vi "Metronome.vi"() -> ()   [LabVIEW 2011, in "Messenging.lvlib" / "Metronome.lvclass"]
uses:
  Metronome.lvclass
  Parallel Process.lvclass
  Interprocess Messenger/TextVarientMessage/MSG.lvclass
  Interprocess Messenger/Receiver/MGR (Receive type).lvclass
  ObserverRegister/ObserverRegistry.lvclass
  Interprocess Messenger/TextVarientMessage/Write (no data).vi
  Interprocess Messenger/TextVarientMessage/Write VarMessage.vi
  Interprocess Messenger/VarMessage/VarMessage.lvclass
panel:
  in  "Startup Message":refnum<class "MSG.lvclass">
  # "QueueMessenger Based"
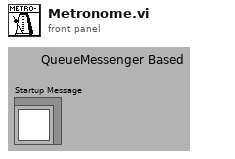
[diagram p1: front panel]
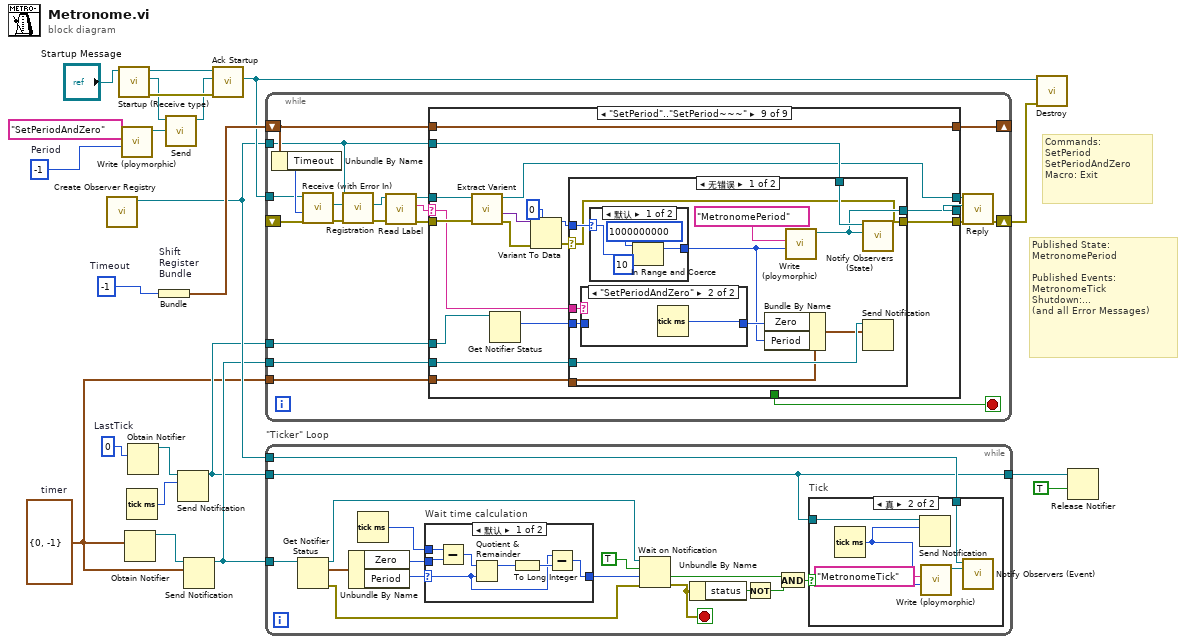
[diagram p0: block diagram]
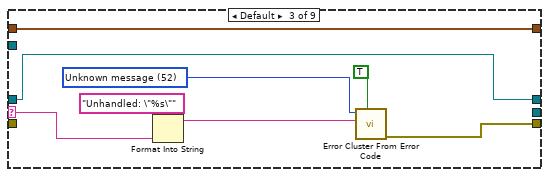
[diagram p6: hidden frame]
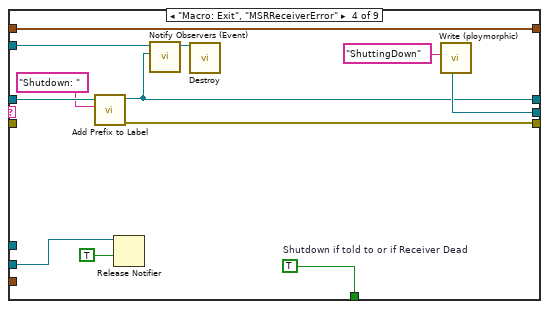
[diagram p7: hidden frame]
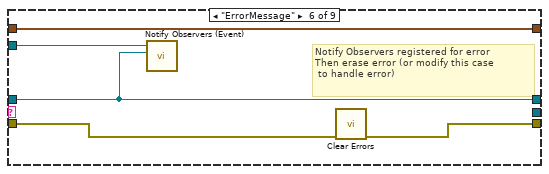
[diagram p9: hidden frame]
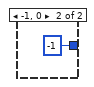
[diagram p12: hidden frame]
diagram:
  w2 = -1  # Period
  w11 = u32 0  # LastTick
  w4 = cluster{"Zero":u32, "Period":i32} {"Zero"=0, "Period"=-1}  # timer
  w19 = -1  # Timeout
  # "Published State:\nMetronomePeriod\n\nPublished Events:\nMetronomeTick\nShutdown:...\n(and all Error Messages)"
  # "Commands:\nSetPeriod\nSetPeriodAndZero\nMacro: Exit"
  n1 = call "Create Observer Registry.vi"() -> ("ObsReg"=w14:refnum<class "ObserverRegistry.lvclass">)  [unwired: 1 in, 10 out]
  n2 = call "Startup (Receive type).vi"("Startup Message"="Startup Message") -> ("error out"=w17:errorcluster, "Command Messenger out"=w6:refnum<class "MGR (Receive type).lvclass">, "Starup Message"=w22:refnum<class "MSG.lvclass">)  [unwired: 1 in, 7 out]
  n3 = call-poly "Write (ploymorphic).vi"("Varient"=w2, "Label"="SetPeriodAndZero") -> ("Message"=w1:refnum<class "VarMessage.lvclass">)  [unwired: 1 in, 8 out]
  n4 = Obtain Notifier(notification data type=w4) -> (notifier out=w15:refnum<notifier>)  [unwired: 2 in, 3 out]
  n5 = Tick Count (ms)() -> (millisecond timer value=w7:u32)
  n6 = Obtain Notifier(notification data type=w11) -> (notifier out=w12:refnum<notifier>)  [unwired: 2 in, 3 out]
  n7 = Bundle "Shift\nRegister\nBundle"("Timeout"=w19) -> (w18:cluster{"Timeout":i32})  [unwired: 1 in]
  n8 = call-dynamic "Send.vi"("Message"=w1, "MSR Parent in"=w6) -> ("MSR Parent out"=w5:refnum<class "MGR (Receive type).lvclass">)  [unwired: 1 in, 8 out]
  n9 = Send Notification(notification=w7, notifier=w12) -> (notifier out=w10:refnum<notifier>)  [unwired: 1 in, 1 out]
  n10 = Send Notification(notification=w4, notifier=w15) -> (notifier out=w13:refnum<notifier>)  [unwired: 1 in, 1 out]
  n11 = call "Ack Startup.vi"("error in"=w17, "Command Messenger"=w5, "Starup Message"=w22) -> ("Command Messenger"=w16:refnum<class "MGR (Receive type).lvclass">)  [unwired: 3 in, 5 out]
  n12 = while {
    shift-right: [w40] -> w20
    shift-left: _ -> [w43]
    shift-right: [w36] -> _
    shift-left: w18 -> [w35]
    tunnel: w16 -> [w34]
    tunnel: w14 -> [w26]
    tunnel: w13 -> [w24]
    tunnel: w10 -> [w25]
    tunnel: w4 -> [w23]
    stop <- w38 stop-if-true
    n13 = Unbundle By Name(w35) -> ("Timeout"=w37:i32)
    n14 = call-dynamic "Receive (with Error In).vi"("error in (no error)"=w43, "timeout in ms (5000)"=w37, "MGR in"=w34) -> ("error out"=w28:errorcluster, "Message"=w33:refnum<class "MSG.lvclass">)  [unwired: 7 out]
    n15 = call "Registration.vi"("error in (no error)"=w28, "Message"=w33, "ObserverRegistry in"=w26) -> ("error out"=w27:errorcluster, "Message (Register Commands filtered out)"=w32:refnum<class "MSG.lvclass">)  [unwired: 7 out]
    n16 = call-dynamic "Read Label.vi"("error in (no error)"=w27, "Message"=w32) -> ("error out"=w29:errorcluster, "Label"=w31:string, "Message"=w30:refnum<class "MSG.lvclass">)  [unwired: 7 out]
    n17 = case shown="\"SetPeriod\"..\"SetPeriod~~~\"" w31 {
      selector: w31 -> [_ _ w57 _ _ _ _ _ w86]
      tunnel: [w45 w47 w50 w60 w71 w73 w78 w81 w84] -> w39
      tunnel: [w44 w48 w51 w61 w70 w75 w79 w82 w89] -> w42
      tunnel: [_ _ _ w64 _ _ _ _ w90] -> w41
      tunnel: [_ _ _ w68 _ _ _ _ _] -> w38
      tunnel: [w46 w49 w52 w69 w72 w77 w80 w83 w92] -> w36
      tunnel: w35 -> [w46 w49 w52 w69 w72 w77 w80 w83 w92]
      tunnel: w30 -> [w44 w48 w51 w63 w70 w75 w79 w82 w97]
      tunnel: w29 -> [w45 w47 _ _ w71 w74 w78 w81 w96]
      tunnel: w26 -> [_ _ _ w66 _ w76 _ _ w91]
      tunnel: w25 -> [_ _ _ _ _ _ _ _ w94]
      tunnel: w24 -> [_ _ _ w58 _ _ _ _ w88]
      tunnel: w23 -> [_ _ _ _ _ _ _ _ w87]
      frame "------- Core (don't modify) --------" {
        # "Core Cases for template"
      }
      frame "<null> message (ignore)", "MSG" {
        # "\"Null\" Message --> Ignore these"
      }
      frame Default {
        w54 = 52 items=["No error", "Argument error", "Memory is full", "Out of zone", "End of file", "File already open", "Generic file I/O error", "File not found", "File permission error", "Disk is full", "Duplicate path", "Too many files open", "System feature not enabled", "Resource file not found", "Cannot add resource", "Resource not found", "Image not found", "Image memory error", "Pen does not exist", "Config type invalid", "Config token not found", "Config parse error", "Config memory error", "Bad external code format", "Bad external code offset", "External code not present", "Null window", "Destroy window error", "Null menu", "Print aborted", "Bad print record", "Print driver error", "Windows error during printing", "Memory error during printing", "Print dialog error", "Generic print error", "Invalid device refnum", "Device not found", "Device parameter error", "Device unit error", "Cannot open device", "Device call aborted", "Generic error", "Cancelled by user", "Object ID too low", "Object ID too high", "Object not in heap", "Unknown heap", "Unknown object (invalid DefProc)", "Unknown object (DefProc not in table)", "Message out of range", "Invalid (null) method", "Unknown message", "Manager call not supported", "Bad address", "Network operation in progress", "Network operation timed out", "Connection is busy", "Network attribute not supported", "Network error", "Address in use", "System out of memory", "Connection aborted", "Connection refused", "Not connected", "Already connected", "Connection closed", "Initialization error (interapplication manager)", "Bad occurrence", "Wait on unbound occurrence handler", "Occurrence queue overflow", "Datalog type conflict", "Unused", "Unrecognized type (interapplication manager)", "Memory corrupt", "Failed to make temporary DLL", "Old CIN version", "Drag socket not found", "Failed to load drop-object", "Failed to register OLE object", "Failed to release OLE object", "Format specifier type mismatch", "Unknown format specifier", "Too few format specifiers", "Too many format specifiers", "Scan failed", "Newer CIN version", "Error converting to variant", "Runtime menu error", "Password tampered", "Variant attribute not found", "Incompatible variant data type", "Event data is not available", "Event Store is not present", "Occurrence is not found", "Event Queue is not created", "Event info is not available", "Refnum passed is NULL", "Error retrieving Class GUID", "Error retrieving CoClass GUID", "Error retrieving TypeLib GUID.", "Bad built application magic bytes.", "Specific driver is different from the specific driver associated with the Logical Name.", "There is no session opened to the class driver.", "Max Error", "MAX - Error with config objects", "MAX - Error loading configuration", "MAX - Group not supported"]
        n18 = Format Into String(format string="Unhandled: \"%s\"", w57) -> (resulting string=w55:string)  [unwired: 2 in, 1 out]
        n19 = call <vilib>:"Error Cluster From Error Code.vi"("show call chain? (False)"=TRUE, "error message (\"\")"=w55, "error code (0)"=w54) -> ("error out"=w50:errorcluster)  [unwired: 1 in, 5 out]
      }
      frame "Macro: Exit", "MSRReceiverError" {
        w68 = TRUE  # Shutdown if told to or if Receiver Dead
        n20 = call-dynamic "Add Prefix to Label.vi"("Prefix to add"="Shutdown: ", "Message"=w63) -> ("error out"=w60:errorcluster, "Message"=w61:refnum<class "MSG.lvclass">)  [unwired: 1 in, 7 out]
        n21 = Release Notifier(notifier=w58, force destroy? (F)=TRUE) -> ()  [unwired: 1 in, 3 out]
        n22 = call "Notify Observers (Event).vi"("Message"=w61, "ObserverRegistry in"=w66) -> ("ObserverRegistry out"=w67:refnum<class "ObserverRegistry.lvclass">)  [unwired: 1 in, 8 out]
        n23 = call "Destroy.vi"("ObserverRegistry.lvclass in"=w67) -> ()  [unwired: 1 in, 10 out]
        n24 = call-poly "Write (ploymorphic).vi"("Label"="ShuttingDown") -> ("Message"=w64:refnum<class "MSG.lvclass">)  [unwired: 1 in, 9 out]
      }
      frame "-------- Core (modify to suit) -----" {
        # "Core Cases for template"
      }
      frame "ErrorMessage" {
        # "Notify Observers registered for error\nThen erase error (or modify this case\n to handle error)"
        n25 = call "Notify Observers (Event).vi"("Message"=w75, "ObserverRegistry in"=w76) -> ()  [unwired: 1 in, 9 out]
        n26 = call <vilib>:"Clear Errors.vi"("error in (no error)"=w74) -> ("error out"=w73:errorcluster)  [unwired: 6 out]
      }
      frame "MSRReceiveTimedOut" {
      }
      frame "-------- Metronome --------" {
      }
      frame "SetPeriod".."SetPeriod~~~" {
        n27 = call-dynamic "Extract Varient.vi"("error in (no error)"=w96, "Message"=w97) -> ("error out"=w99:errorcluster, "Varient"=w98:variant, "Message"=w89:refnum<class "MSG.lvclass">)  [unwired: 1 in, 6 out]
        n28 = Get Notifier Status(notifier=w94) -> (current notification=w93:u32)  [unwired: 1 in, 4 out]
        n29 = Variant To Data(error in=w99, type=0 ("Period"), Variant=w98) -> (data=w100:i32, error out=w85:errorcluster)
        n30 = case shown="无错误" w85 {
          selector: w85 -> [w101 w120]
          tunnel: w100 -> [w112 _]
          tunnel: w93 -> [w108 _]
          tunnel: w91 -> [w107 _]
          tunnel: [w106 _] -> w90
          tunnel: w88 -> [w105 _]
          tunnel: w87 -> [w103 _]
          tunnel: w86 -> [w102 _]
          tunnel: [w101 w120] -> w84
          frame No Error {
            n31 = case shown="\"SetPeriodAndZero\"" w102 {
              tunnel: w108 -> [w118 _]
              tunnel: [w118 w119] -> w111
              frame "SetPeriod", Default {
              }
              frame "SetPeriodAndZero" {
                n32 = Tick Count (ms)() -> (millisecond timer value=w119:u32)
              }
            }
            n33 = case shown="默认" w112 {
              selector: w112 -> [w113 _]
              tunnel: [w114 -1 ("upper limit")] -> w110
              frame Default {
                n34 = In Range and Coerce(upper limit=1000000000, x=w113, lower limit=10) -> (coerced(x)=w114:i32)  [unwired: 1 out]
              }
              frame -1, 0 {
              }
            }
            n35 = Bundle By Name(cluster=w103, "Zero"=w111, "Period"=w110) -> (w104:cluster{"Zero":u32, "Period":i32})
            n36 = call-poly "Write (ploymorphic).vi"("Varient"=w110, "Label"="MetronomePeriod") -> ("Message"=w106:refnum<class "VarMessage.lvclass">)  [unwired: 1 in, 8 out]
            n37 = call "Notify Observers (State).vi"("State Message"=w106, "ObserverRegistry in"=w107) -> ()  [unwired: 1 in, 9 out]
            n38 = Send Notification(notification=w104, notifier=w105) -> ()  [unwired: 1 in, 2 out]
          }
          frame Error {
          }
        }
      }
    }
    n39 = call-dynamic "Reply.vi"("error in (no error)"=w39, "Reply"=w41, "Message to Reply to"=w42) -> ("error out"=w40:errorcluster)  [unwired: 8 out]
  }
  n40 = while "\"Ticker\" Loop" {
    tunnel: w13 -> [w131]
    tunnel: w14 -> [w122]
    tunnel: w10 -> [w121]
    tunnel: [w121] -> w8
    stop <- w125 stop-if-true
    n41 = Get Notifier Status(notifier=w131) -> (notifier out=w130:refnum<notifier>, current notification=w129:cluster{"Zero":u32, "Period":i32}, error out=w127:errorcluster)  [unwired: 1 in, 2 out]
    n42 = Unbundle By Name(w129) -> ("Zero"=w136:u32, "Period"=w134:i32)
    n43 = Tick Count (ms)() -> (millisecond timer value=w135:u32)
    n44 = case "Wait time calculation" shown="默认" w134 {
      selector: w134 -> [w142 w149]
      tunnel: [w144 w149] -> w128
      tunnel: w136 -> [w148 _]
      tunnel: w135 -> [w147 _]
      frame Default {
        n45 = Subtract(x=w147, y=w148) -> (x-y=w146:u32)
        n46 = Quotient & Remainder(x=w146, y=w142) -> (x-y*floor(x/y)=w145:u32)  [unwired: 1 out]
        n47 = To Long Integer(number=w145) -> (32bit integer=w143:i32)
        n48 = Subtract(x=w142, y=w143) -> (x-y=w144:i32)
      }
      frame -1 {
      }
    }
    n49 = Wait on Notification(notifier=w130, ignore previous (F)=TRUE, timeout in ms (-1)=w128, error in (no error)=w127) -> (timed out?=w132:bool, error out=w125:errorcluster)  [unwired: 2 out]
    n50 = Unbundle By Name(w125) -> ("status"=w123:bool)
    n51 = Not(x=w123) -> (.not. x?=w124:bool)
    n52 = And(x=w132, y=w124) -> (x .and. y?=w126:bool)
    n53 = case "Tick" shown="真" w126 {
      tunnel: w122 -> [_ w139]
      tunnel: w121 -> [_ w138]
      frame False {
      }
      frame True {
        n54 = Tick Count (ms)() -> (millisecond timer value=w137:u32)
        n55 = Send Notification(notification=w137, notifier=w138) -> ()  [unwired: 1 in, 2 out]
        n56 = call-poly "Write (ploymorphic).vi"("Varient"=w137, "Label"="MetronomeTick") -> ("Message"=w140:refnum<class "VarMessage.lvclass">)  [unwired: 1 in, 8 out]
        n57 = call "Notify Observers (Event).vi"("Message"=w140, "ObserverRegistry in"=w139) -> ()  [unwired: 1 in, 9 out]
      }
    }
  }
  n58 = call-dynamic "Destroy.vi"("error in (no error)"=w20, "Messenger in"=w16) -> ()  [unwired: 10 out]
  n59 = Release Notifier(notifier=w8, force destroy? (F)=TRUE) -> ()  [unwired: 1 in, 3 out]
